vi "ConvertFESTOOutputBytes.vi"(10 "Festo Block":u8, 11 "Valves":bool[](array[boolean])) -> (3 "Bytes":u8[](array[numeric]))   [LabVIEW 2011]
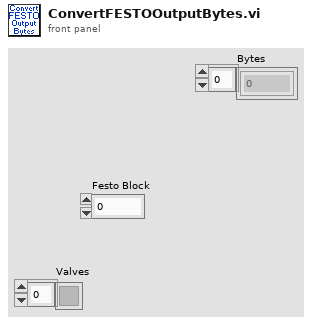
[diagram p1: front panel]
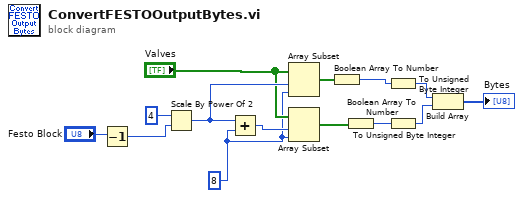
[diagram p0: block diagram]
diagram:
  w10 = u8 8 ("y")
  n1 = Decrement(x="Festo Block") -> (x-1=w6:u8)
  n2 = Scale By Power Of 2(n=4, x=w6) -> (x*2^n=w13:u8)
  n3 = Add(x=w13, y=w10) -> (x+y=w11:u8)
  n4 = Array Subset(array="Valves", index=w13, length=w10) -> (w9:bool[])
  n5 = Array Subset(array="Valves", index=w11, length=w10) -> (w8:bool[])
  n6 = Boolean Array To Number(Boolean array=w9) -> (number=w4:u32)
  n7 = Boolean Array To Number(Boolean array=w8) -> (number=w5:u32)
  n8 = To Unsigned Byte Integer(number=w4) -> (unsigned 8bit integer=w2:u8)
  n9 = To Unsigned Byte Integer(number=w5) -> (unsigned 8bit integer=w3:u8)
  n10 = Build Array(w2, w3) -> (→"Bytes":u8[])
